vi "Main.vi"() -> ()   [LabVIEW 2016]
doc: "--\nCopyright © 2017 Composed SystemsI All rights reserved.\n\nAuthor: Jon McBee <jon.mcbee@composed.io>\n\nThis library is provided \"AS IS\" ,WITHOUT WARRANTIES OR\nCONDITIONS OF ANY KIND, either express or implied.\n\nComposed Systems -- composed.io\n\nStream 0.0.1.1\nJon McBee - Composed Systems\nCopyright (c) 2017, Composed Systems"
uses:
  <vilib>/Composed Systems/Stream/Sandbox/Async Actor Test/Parrot Actor/Parrot.lvclass
  D:/Repos/Stream/software/Mediator/Classes/Mediated Asynchronous Actor/Mediated Asynchronous Actor.lvclass
  <vilib>/Composed Systems/Stream/Mediator/Classes/Message Broker Interface Ref/Message Broker Interface Ref.lvclass
  D:/Repos/Stream/software/Mediator/Classes/Message Broker Interface/Message Broker Interface.lvclass
  <vilib>/Composed Systems/Stream/Mediator/Classes/Message Transport Queue/Message Transport Queue.lvclass
  D:/Repos/Stream/software/Mediator/Classes/Message Transport Interface/Message Transport Interface.lvclass
  <vilib>/Composed Systems/Stream/Mediator/Classes/Message Transport Binding/Message Transport Binding.lvclass
  <vilib>/Composed Systems/Stream/Mediator/Classes/Mediated Asynchronous Actor/Mediated Asynchronous Actor.lvclass
  <vilib>/Composed Systems/Stream/Sandbox/Async Actor Test/Parrot Msg/Parrot Msg.lvclass
  <vilib>/Composed Systems/Stream/Mediator/Classes/Message Command Stop/Stop Msg.lvclass
panel:
  in  "Send":bool
  out "Rx String":string
  in  "Tx String":string
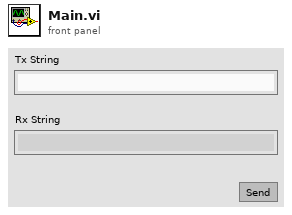
[diagram p1: front panel]
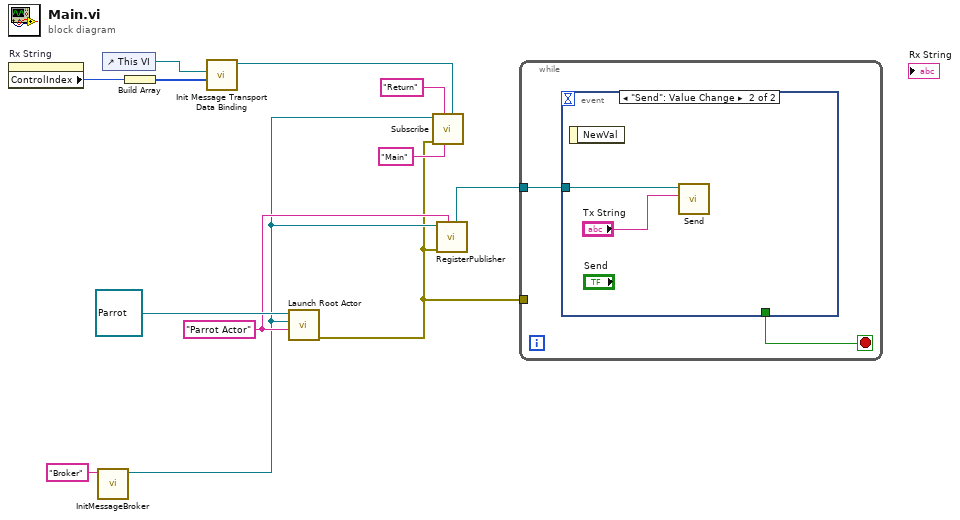
[diagram p0: block diagram]
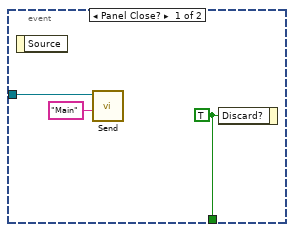
[diagram p2: hidden frame]
diagram:
  w10 = "Parrot Actor" ("Actor Name")
  n1 = property on="Rx String" class="Str"() -> ("ControlIndex"=w8:i32)  [unwired: 2 in, 2 out]
  n2 = call <vilib>:"InitMessageBroker.vi"("Broker Name"="Broker") -> ("Message Broker Interface Ref out"=w2:refnum<class "Message Broker Interface Ref.lvclass">)  [unwired: 9 in, 1 out]
  n3 = control-ref of="This VI"() -> (w6:refnum<vi>)
  n4 = Build Array(w8) -> (w7:i32[])
  n5 = call <vilib>:"Init Message Transport Data Binding.vi"("Control Indexes"=w7, "VI Refnum"=w6) -> ("Message Transport Binding out"=w5:refnum<class "Message Transport Binding.lvclass">)  [unwired: 8 in, 1 out]
  n6 = call <vilib>:"Launch Root Actor.vi"("Actor Name"=w10, "Message Broker"=w2, "Mediated Asynchronous Actor in"=refnum<class "Parrot.lvclass"> refnum ("Parrot.lvclass")) -> ("error out"=w1:errorcluster)  [unwired: 7 in, 1 out]
  n7 = call-dynamic "Subscribe.vi"("Message Transport Interface"=w5, "Subscriber Name"="Main", "Topic Name"="Return", "error in (no error)"=w1, "Message Broker Interface TAP in"=w2) -> ()  [unwired: 4 in, 3 out]
  n8 = call-dynamic "RegisterPublisher.vi"("Topic Name"=w10, "error in (no error)"=w1, "Message Broker Interface Ref in"=w2) -> ("Transport"=w9:refnum<class "Message Transport Queue.lvclass">)  [unwired: 4 in, 4 out]
  n9 = while {
    tunnel: w1 -> [_]
    tunnel: w9 -> [w14]
    stop <- w13 stop-if-true
    n10 = event shown="[1] \"Send\": Value Change" {
      selector: _ -> [_ _]
      dyn-events: _ -> [_ _]
      timeout: _ -> [_ _]
      tunnel: w14 -> [w16 w19]
      tunnel: [w17 _] -> w13
      event Panel Close? {
        w17 = TRUE ("Discard?")
        n11 = event-data() -> ()  [unwired: 1 in, 1 out]
        n12 = call <vilib>:"Send.vi"("Caller Actor Name"="Main", "Message Transport"=w16) -> ()  [unwired: 9 in, 1 out]
        n13 = event-data("Discard?"=w17) -> ()  [unwired: 1 in, 1 out]
      }
      event "Send": Value Change {
        n14 = event-data() -> ()  [unwired: 1 in, 1 out]
        n15 = call <vilib>:"Send.vi"("Tx String"="Tx String", "Message Transport Queue in"=w19) -> ()  [unwired: 9 in, 1 out]
      }
    }
  }
